vi "CVT Session FGV.vi"(7 "State":enum16{"Init", "Get"}(ring)=enum."Get", 11 "CVT Session":refnum<data-value>) -> (3 "CVT Session Out":refnum<data-value>)   [LabVIEW 2014, in "Controller.lvlib" / "Controller.lvclass"]
uses:
  Controller.lvclass
  <userlib>/_Session Fwk/Session - Root.lvclass
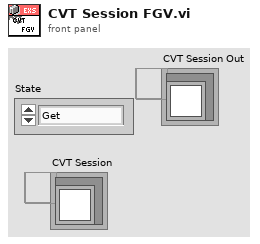
[diagram p1: front panel]
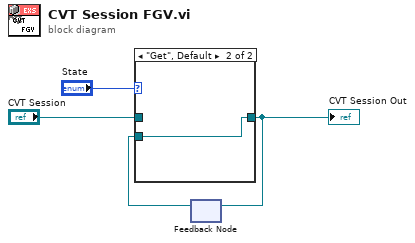
[diagram p0: block diagram]
diagram:
  n1 = feedback #1() -> (w3:refnum<data-value>)  [unwired: 1 in]
  n2 = case shown="\"Get\", Default" "State" {
    tunnel: "CVT Session" -> [w5 _]
    tunnel: [w5 w6] -> w1
    tunnel: w3 -> [_ w6]
    frame "Init" {
    }
    frame "Get", Default {
    }
  }
  "CVT Session Out" <- w1
  n3 = feedback-in #1(w1) -> ()
